vi "温度校准.vi"(7 "校准参数":u16(ring) caption="校准参数：" items=["pH", "DO", "浊度", "电导率", "叶绿素a", "藻密度", "ORP", "DO2"], 8 "error in (no error)":errorcluster caption="错误输入（无错误）", 11 "校准温度":sgl) -> (0 "error out":errorcluster caption="错误输出")   [LabVIEW 2016, in "斯坦道多参数.lvlib"]
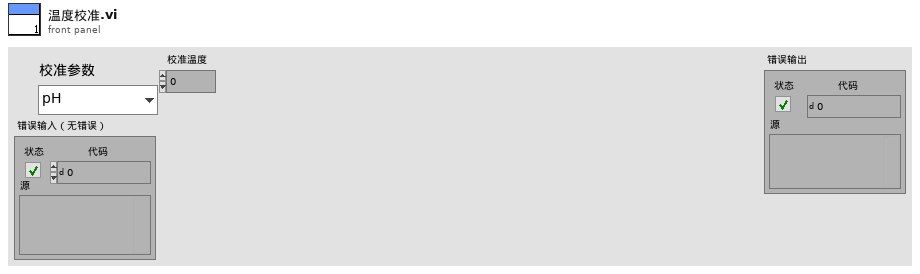
[diagram p1: front panel]
types:
  T1 = enum16{"NULL", "pH", "Cond", "DO", "Turb", "ORP"}
  T2 = enum16{"null", "pH", "DO", "浊度", "电导率", "叶绿素a", "藻密度"}
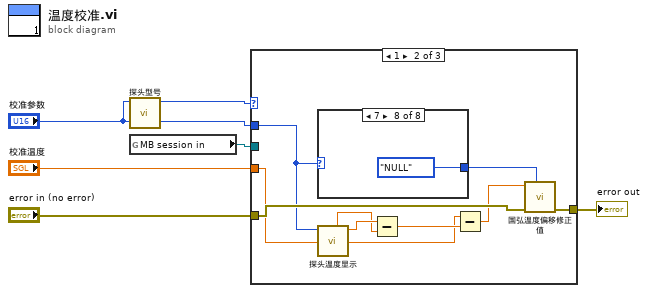
[diagram p0: block diagram]
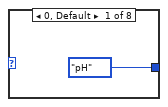
[diagram p3: hidden frame]
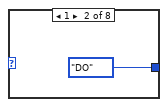
[diagram p4: hidden frame]
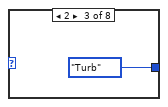
[diagram p5: hidden frame]
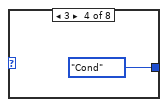
[diagram p6: hidden frame]
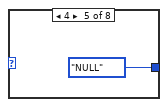
[diagram p7: hidden frame]
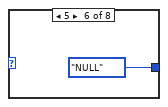
[diagram p8: hidden frame]
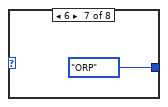
[diagram p9: hidden frame]
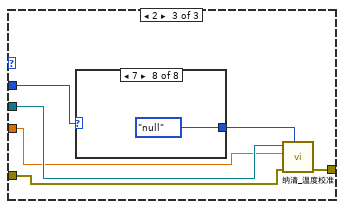
[diagram p10: hidden frame]
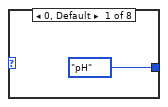
[diagram p11: hidden frame]
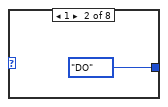
[diagram p12: hidden frame]
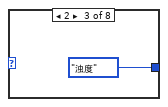
[diagram p13: hidden frame]
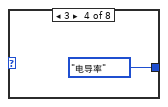
[diagram p14: hidden frame]
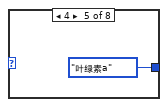
[diagram p15: hidden frame]
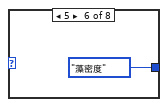
[diagram p16: hidden frame]
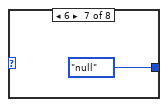
[diagram p17: hidden frame]
diagram:
  n1 = call "探头型号.vi"("校准参数"="校准参数") -> ("探头型号"=w6:u16)  [unwired: 8 in, 2 out]
  n2 = global read "多参数全局变量.vi" "MB session in"() -> (w4:refnum<class "MB_Master.lvclass">)
  n3 = case shown="1" w6 {
    tunnel: "校准参数" -> [_ w13 w26]
    tunnel: w4 -> [_ _ w28]
    tunnel: "error in (no error)" -> [w7 w16 w30]
    tunnel: [w7 w15 w29] -> w2
    tunnel: "校准温度" -> [_ w9 w27]
    frame 0, Default {
    }
    frame 1 {
      n4 = case shown="7" w13 {
        tunnel: [T1."pH" ("探头") T1."DO" ("探头") T1."Turb" ("探头") T1."Cond" ("探头") T1."NULL" ("探头") T1."NULL" ("探头") T1."ORP" ("探头") T1."NULL" ("探头")] -> w14
        frame 0, Default {
        }
        frame 1 {
        }
        frame 2 {
        }
        frame 3 {
        }
        frame 4 {
        }
        frame 5 {
        }
        frame 6 {
        }
        frame 7 {
        }
      }
      n5 = call "探头温度显示.vi"("校准参数"=w13) -> ("温度数据"=w12:sgl, "温度偏移修正值"=w11:sgl)  [unwired: 9 in]
      n6 = Subtract(x=w12, y=w11) -> (x-y=w10:sgl)
      n7 = Subtract(x=w9, y=w10) -> (x-y=w8:sgl)
      n8 = call "国弘温度偏移修正值.vi"("探头"=w14, "error in (no error)"=w16, "温度偏移修正值"=w8) -> ("error out"=w15:errorcluster)  [unwired: 7 in, 1 out]
    }
    frame 2 {
      n9 = case shown="7" w26 {
        tunnel: [T2."pH" ("探头") T2."DO" ("探头") T2."浊度" ("探头") T2."电导率" ("探头") T2."叶绿素a" ("探头") T2."藻密度" ("探头") T2."null" ("探头") T2."null" ("探头")] -> w25
        frame 0, Default {
        }
        frame 1 {
        }
        frame 2 {
        }
        frame 3 {
        }
        frame 4 {
        }
        frame 5 {
        }
        frame 6 {
        }
        frame 7 {
        }
      }
      n10 = call "纳清_温度校准.vi"("探头"=w25, "error in (no error)"=w30, "校准温度"=w27, "MB session in"=w28) -> ("error out"=w29:errorcluster)  [unwired: 6 in, 1 out]
    }
  }
  "error out" <- w2
